vi "DownSampleAndShiftiRF (SubVI).vi"(7 "Normalize? (T)":bool=TRUE, 10 "PeakIndex (250)":i32=250, 11 "ArrayIn":dbl[](array[numeric])) -> (3 "ArrayOut":dbl[](array[numeric]))   [LabVIEW 2024]
uses:
  <vilib>/Analysis/baseanly.llb/Mean (DBL).vi
  <vilib>/Analysis/NI_AALBase.lvlib
panel:
  out "Waveform Graph":dbl[](graph)
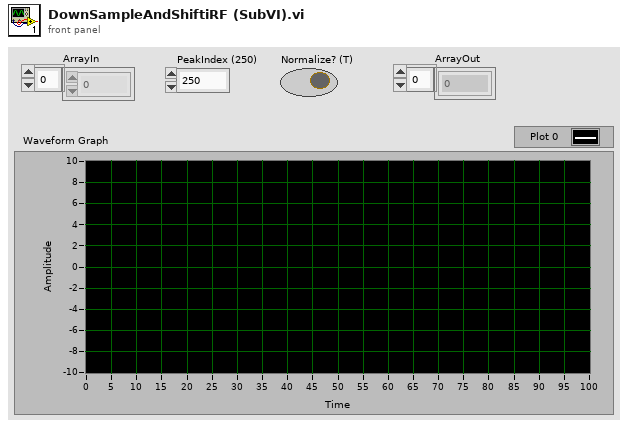
[diagram p1: front panel]
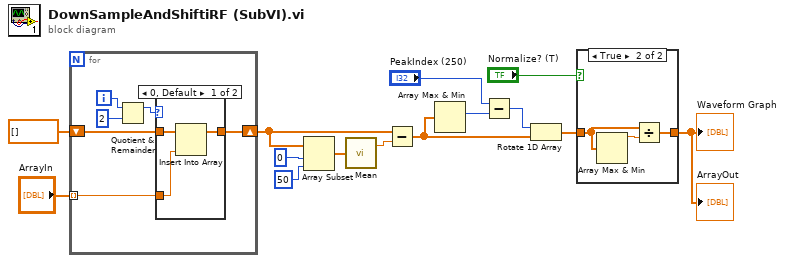
[diagram p0: block diagram]
diagram:
  n1 = for {
    tunnel: "ArrayIn" -> [w16] mode=indexing
    shift-right: [w15] -> w9
    shift-left: dbl[] [] -> [w17]
    i -> [w20]
    n2 = Quotient & Remainder(x=w20, y=2) -> (x-y*floor(x/y)=w18:i32)  [unwired: 1 out]
    n3 = case shown="0, Default" w18 {
      tunnel: w17 -> [w23 w24]
      tunnel: w16 -> [w22 _]
      tunnel: [w21 w24] -> w15
      frame 0, Default {
        n4 = Insert Into Array(array=w23, new element=w22) -> (w21:dbl[])  [unwired: 1 in]
      }
      frame 1 {
      }
    }
  }
  n5 = Array Subset(array=w9, index=0, length=50) -> (w10:dbl[])
  n6 = call-poly <vilib>:"Mean.vi"("X"=w10) -> ("mean"=w8:dbl)  [unwired: 1 out]
  n7 = Subtract(x=w9, y=w8) -> (x-y=w5:dbl[])
  n8 = Array Max & Min(array=w5) -> (max index (indices)=w7:i32)  [unwired: 3 out]
  n9 = Subtract(x="PeakIndex (250)", y=w7) -> (x-y=w4:i32)
  n10 = Rotate 1D Array(1:w5, 2:w4) -> (0:w2:dbl[])
  n11 = case shown="True" "Normalize? (T)" {
    tunnel: w2 -> [w25 w28]
    tunnel: [w25 w26] -> w1
    frame False {
    }
    frame True {
      n12 = Array Max & Min(array=w28) -> (max value=w27:dbl)  [unwired: 3 out]
      n13 = Divide(x=w28, y=w27) -> (x/y=w26:dbl[])
    }
  }
  "ArrayOut" <- w1
  "Waveform Graph" <- w1
